vi "Get Hi Leaf Wet Alarm V.vi"(8 "error in (no error)":errorcluster, 11 "sensorNumber":i16) -> (0 "error out":errorcluster, 3 "function return":sgl)   [LabVIEW 2009, in "VantagePro.lvlib"]
doc: "DllAccess float _stdcall GetHiLeafWetAlarm_V(short sensorNumber);"
uses:
  VantagePro.lvlib
  <userlib>/VantagePro/VantagePro.dll
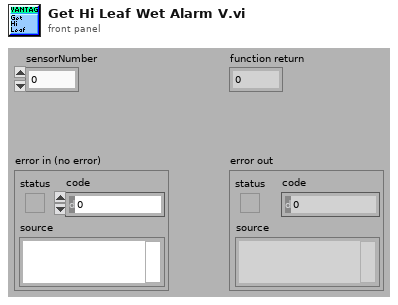
[diagram p1: front panel]
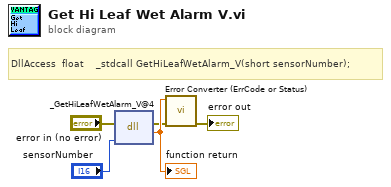
[diagram p0: block diagram]
diagram:
  # "DllAccess  float    _stdcall GetHiLeafWetAlarm_V(short sensorNumber);"
  n1 = dll-call lib="C:/Program Files/National Instruments/LabVIEW 2010/user.lib/VantagePro/VantagePro.*" fn="_GetHiLeafWetAlarm_V@4"(error in="error in (no error)", "sensorNumber"="sensorNumber") -> (error out=w2:errorcluster, w5:sgl)  [unwired: 3 in, 1 out]
  "function return" <- w5
  n2 = call "Error Converter (ErrCode or Status).vi"("error in (no error)"=w2, "error code"=w5) -> ("error out"=→"error out":errorcluster)  [unwired: 9 in]
